vi "Start.vi"(8 "error in (no error)":errorcluster, 9 "Timeout [ms] (-1)":i32=-1, 11 "Process In":refnum<class "Debug Process.lvclass">) -> (0 "error out":errorcluster, 1 "timed out?":bool, 3 "Process Out":refnum<class "Debug Process.lvclass">)   [LabVIEW 2020, in "Debug Process.lvclass"]
doc: "This VI starts the process which runs asyncronously. The VI blocks the execution until the process has reached its' running state, or the specified timeout expires."
uses:
  Debug Process.lvclass
  Debug Process.lvclass/Debug Process.ctl
  Public/Lifecycle/Lifecycle State.ctl
  <vilib>/Utility/error.llb/Clear Errors.vi
  <vilib>/Utility/error.llb/Error Cluster From Error Code.vi
  Private/SubVIs/Process.vi
  <vilib>/ErrorRing/Error Ring.xnode
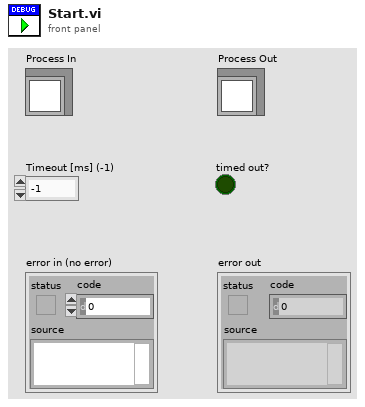
[diagram p1: front panel]
types:
  T1 = typedef "Debug Process.lvclass/Lifecycle State.ctl" = enum16{"Uninitialized", "Initialized", "Started", "Running", "Stopped", "Finished"}
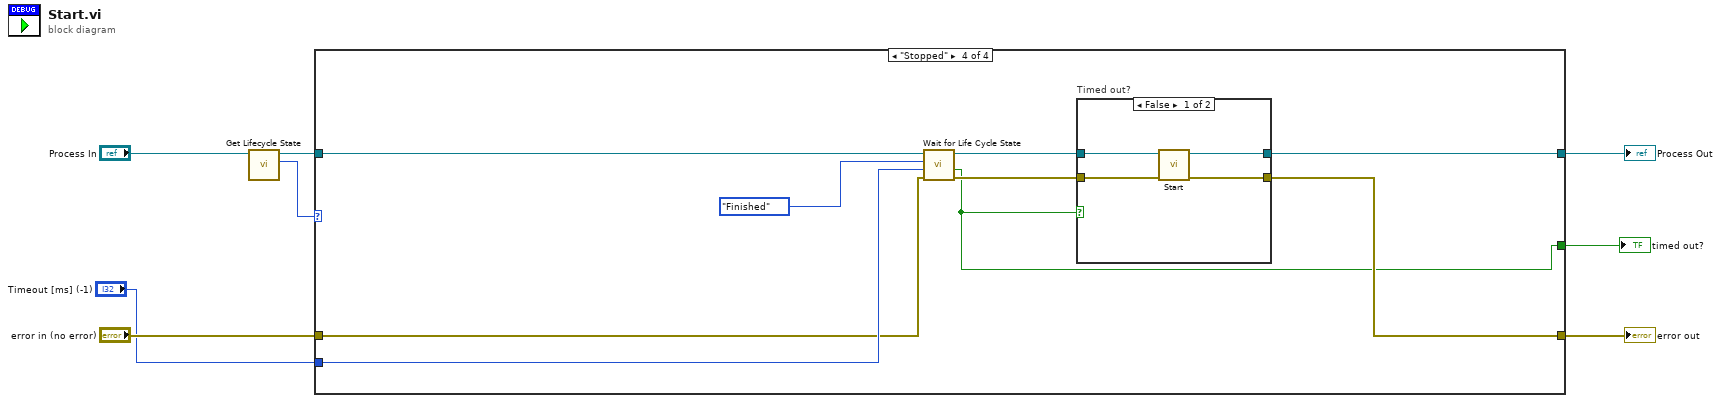
[diagram p0: block diagram]
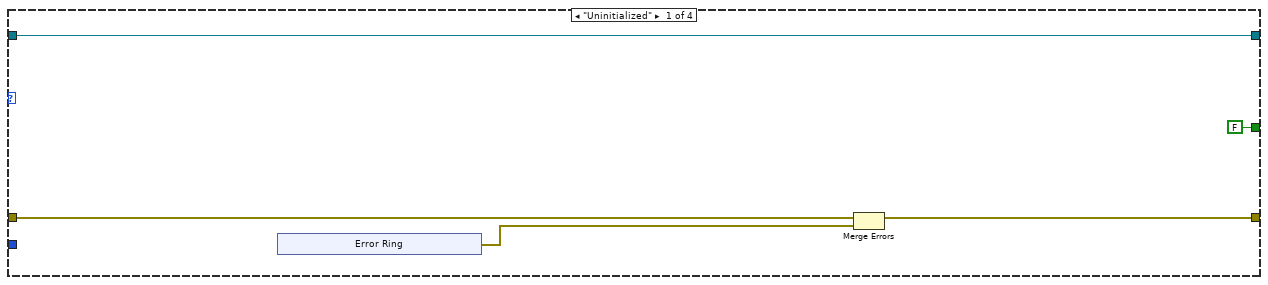
[diagram p2: hidden frame]
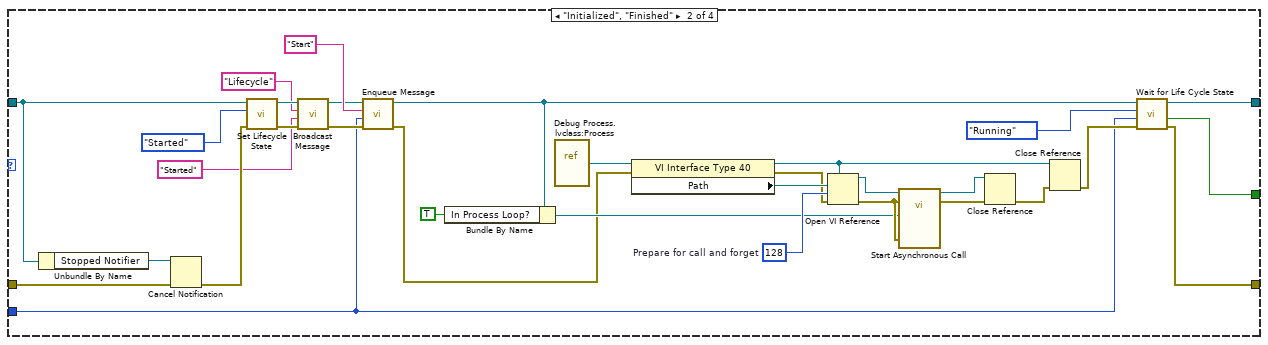
[diagram p3: hidden frame]
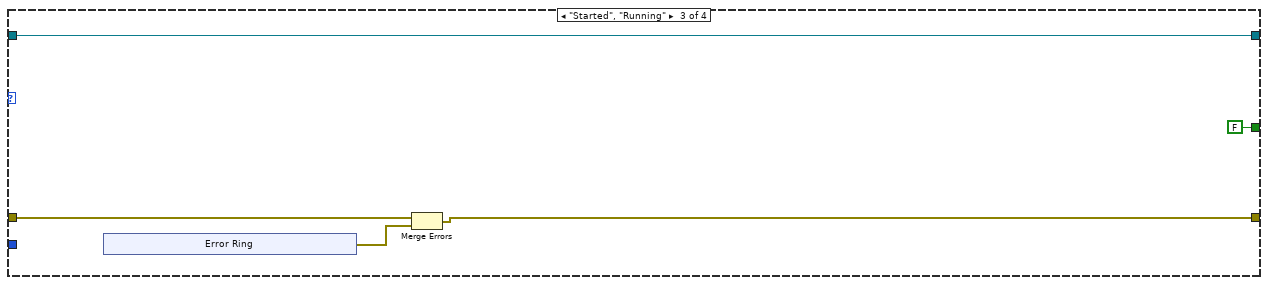
[diagram p4: hidden frame]
diagram:
  n1 = call "Get Lifecycle State.vi"("Process In"="Process In") -> ("Lifecycle State"=w2:T1, "Process Out"=w3:refnum<class "Debug Process.lvclass">)  [unwired: 7 in, 2 out]
  n2 = case shown="\"Stopped\"" w2 {
    tunnel: [w12 w35 w54 w60] -> w7
    tunnel: [w11 w33 w52 w62] -> w6
    tunnel: w3 -> [w12 w38 w54 w67]
    tunnel: "error in (no error)" -> [w10 w41 w51 w64]
    tunnel: "Timeout [ms] (-1)" -> [_ w19 _ w65]
    tunnel: [FALSE ("timed out?") w18 FALSE ("timed out?") w59] -> w1
    frame "Uninitialized" {
      n3 = xnode "Error Ring"() -> ("error out"=w13:errorcluster)
      n4 = Merge Errors(w10, w13) -> (w11:errorcluster)
    }
    frame "Initialized", "Finished" {
      w46 = 128  # Prepare for call and forget
      n5 = Unbundle By Name(w38) -> ("Stopped Notifier"=w42:refnum<notifier>)
      n6 = Cancel Notification(0:w42, 3:w41) -> (11:w31:errorcluster)  [unwired: 2 out]
      n7 = call "Set Lifecycle State.vi"("error in (no error)"=w31, "Lifecycle State"=Lifecycle_State."Started", "Process In"=w38) -> ("error out"=w26:errorcluster, "Process Out"=w24:refnum<class "Debug Process.lvclass">)  [unwired: 7 in]
      n8 = call-dynamic "Broadcast Message.vi"("error in (no error)"=w26, "Message Data"="Started" ("Message"), "Message"="Lifecycle", "Process In"=w24) -> ("error out"=w25:errorcluster, "Process Out"=w23:refnum<class "Debug Process.lvclass">)  [unwired: 6 in]
      n9 = call "Enqueue Message.vi"("error in (no error)"=w25, "Message Data"=w19, "Message"="Start", "Process In"=w23) -> ("error out"=w37:errorcluster, "Process Out"=w34:refnum<class "Debug Process.lvclass">)  [unwired: 6 in]
      n10 = Bundle By Name(cluster=w34, "In Process Loop?"=TRUE) -> (w39:refnum<class "Debug Process.lvclass">)
      n11 = vi-ref "Debug Process.lvclass:Process.vi"() -> (w47:refnum<vi>)
      n12 = property class="VI Interface Type 40"(reference=w47, error in=w37) -> (reference out=w29:refnum<vi>, error out=w30:errorcluster, "Path"=w44:path)
      n13 = Open VI Reference(type specifier VI Refnum (for type only)=w29, vi path=w44, options=w46, error in (no error)=w30) -> (vi reference=w45:refnum<vi>, error out=w43:errorcluster)  [unwired: 2 in]
      n14 = call-by-ref "Start Asynchronous Call"(reference=w45, error in=w43, 8:"error in (no error)"=w43, "Process In"=w39) -> (reference out=w49:refnum<vi>, error out=w48:errorcluster)  [unwired: 8 in, 2 out]
      n15 = Close Reference(reference=w49, error in (no error)=w48) -> (error out=w28:errorcluster)
      n16 = Close Reference(reference=w29, error in (no error)=w28) -> (error out=w27:errorcluster)
      n17 = call "Wait for Life Cycle State.vi"("error in (no error)"=w27, "timeout in ms (-1)"=w19, "Lifecycle State"=Lifecycle_State."Running", "Process In"=w34) -> ("error out"=w33:errorcluster, "timed out?"=w18:bool, "Process Out"=w35:refnum<class "Debug Process.lvclass">)  [unwired: 5 in]
    }
    frame "Started", "Running" {
      n18 = xnode "Error Ring"() -> ("error out"=w53:errorcluster)
      n19 = Merge Errors(w51, w53) -> (w52:errorcluster)
    }
    frame "Stopped" {
      n20 = call "Wait for Life Cycle State.vi"("error in (no error)"=w64, "timeout in ms (-1)"=w65, "Lifecycle State"=Lifecycle_State."Finished", "Process In"=w67) -> ("error out"=w63:errorcluster, "timed out?"=w59:bool, "Process Out"=w61:refnum<class "Debug Process.lvclass">)  [unwired: 5 in]
      n21 = case "Timed out?" shown="False" w59 {
        tunnel: w63 -> [w71 w72]
        tunnel: [w70 w72] -> w62
        tunnel: w61 -> [w69 w73]
        tunnel: [w68 w73] -> w60
        frame False {
          n22 = call "Start.vi"("error in (no error)"=w71, "Process In"=w69) -> ("error out"=w70:errorcluster, "Process Out"=w68:refnum<class "Debug Process.lvclass">)  [unwired: 7 in, 1 out]
        }
        frame True {
        }
      }
    }
  }
  "error out" <- w6
  "Process Out" <- w7
  "timed out?" <- w1
